vi "Control_BIn.vi"(0 "Control_1":T5={"Turbidotato 1"=1.5, "Habilitar T1"=TRUE, "Habilitar T2"=TRUE, "Habilitar T3"=TRUE, "Habilitar T4"=TRUE, "Habilitar T5"=TRUE, "Habilitar T6"=TRUE, "Habilitar T7"=TRUE, "Habilitar T8"=TRUE, "Turbidotato 2"=1.5, "Turbidotato 3"=1.5, "Turbidotato 4"=1.5, "Turbidotato 5"=1.5, "Turbidotato 6"=1.5, "Turbidotato 7"=1.5, "Turbidotato 8"=1.5, "Modo T1"=TRUE, "Modo T2"=TRUE, "Modo T3"=TRUE, "Modo T4"=TRUE, "Modo T5"=TRUE, "Modo T6"=TRUE, "Modo T7"=TRUE, "Modo T8"=TRUE} caption="Control" {"Turbidotato 8" min=0.5 max=1.5 step=0.01; "Turbidotato 7" min=0.5 max=1.5 step=0.01; "Turbidotato 6" min=0.5 max=1.5 step=0.01; "Turbidotato 5" min=0.5 max=1.5 step=0.01; "Turbidotato 4" min=0.5 max=1.5 step=0.01; "Turbidotato 3" min=0.5 max=1.5 step=0.01; "Turbidotato 2" min=0.5 max=1.5 step=0.01; "Turbidotato 1" min=0.5 max=1.5 step=0.01}, 1 "Minimos":dbl[](array[numeric]), 2 "Manual_ON":T4, 3 "Manual_Off":T3, 4 "Tiempos ON":T2={"T.M.CH1"=20, "T.M.CH2"=20, "T.M.CH3"=20, "T.M.CH4"=20, "T.M.CH5"=20, "T.M.CH6"=20, "T.M.CH7"=20, "T.M.CH8"=20} {"T.M.CH8" min=1 step=1; "T.M.CH7" min=1 step=1; "T.M.CH6" min=1 step=1; "T.M.CH5" min=1 step=1; "T.M.CH4" min=1 step=1; "T.M.CH3" min=1 step=1; "T.M.CH2" min=1 step=1; "T.M.CH1" min=1 step=1}, 5 "Tiempos OFF":T1={"T.M.CH1"=20, "T.M.CH2"=20, "T.M.CH3"=20, "T.M.CH4"=20, "T.M.CH5"=20, "T.M.CH6"=20, "T.M.CH7"=20, "T.M.CH8"=20} {"T.M.CH8" min=1 step=1; "T.M.CH7" min=1 step=1; "T.M.CH6" min=1 step=1; "T.M.CH5" min=1 step=1; "T.M.CH4" min=1 step=1; "T.M.CH3" min=1 step=1; "T.M.CH2" min=1 step=1; "T.M.CH1" min=1 step=1}, 6 "Enable Turbi?":bool, 7 "Error In":errorcluster, 8 "T-On (s)":dbl, 10 "T+ (s)":dbl=1.0 min=1.0 max=20.0) -> (20 "Estados":bool[](array[boolean]), 21 "B_OUT":bool, 27 "Error Out":errorcluster)   [LabVIEW 2013]
uses:
  Controles/Control_1_TB.ctl
  Controles/Manual_ON_TB.ctl
  Controles/Manual_OFF_TB.ctl
  Controles/Tiempos_ON_TB.ctl
  Controles/Tiempos_OFF_TB.ctl
panel:
  # "para modo Turbidostato"
  # "MODO TURBIDOSTATO"
  # "T. OFF (s)"
  # "T. ON (s)"
  # "Habilitar"
  # "Modo"
  # "CH 1"
  # "CH 2"
  # "CH 3"
  # "CH 4"
  # "CH 5"
  # "CH 6"
  # "CH 7"
  # "CH 8"
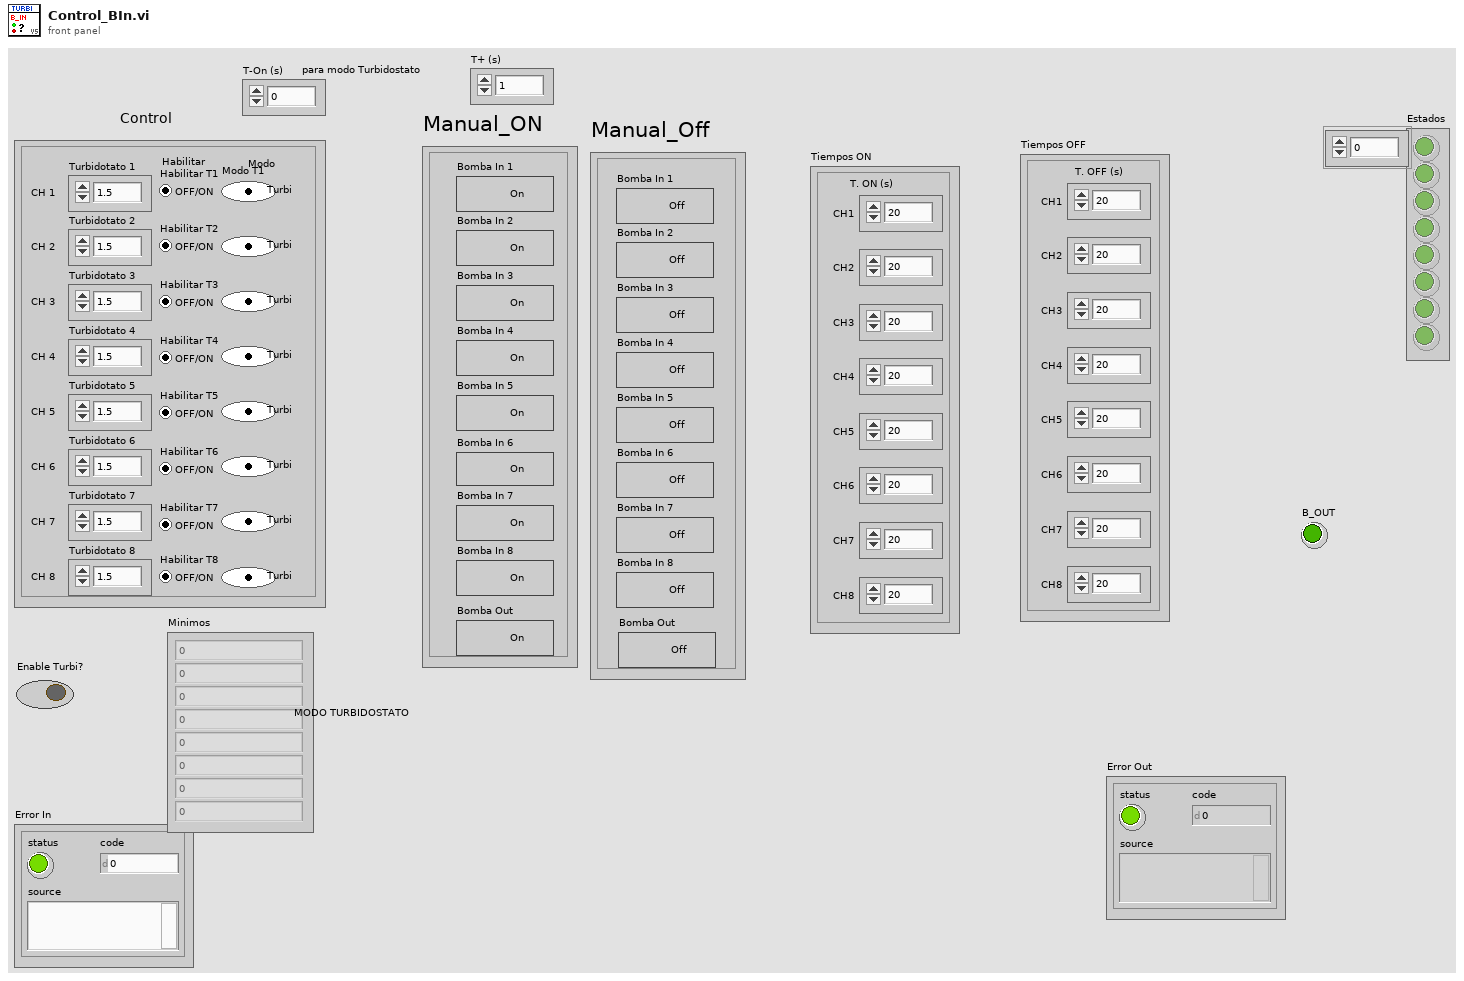
[diagram p1: front panel]
types:
  T1 = typedef "Tiempos_OFF_TB.ctl" = cluster{"T.M.CH1":u16, "T.M.CH2":u16, "T.M.CH3":u16, "T.M.CH4":u16, "T.M.CH5":u16, "T.M.CH6":u16, "T.M.CH7":u16, "T.M.CH8":u16}
  T2 = typedef "Tiempos_ON_TB.ctl" = cluster{"T.M.CH1":u16, "T.M.CH2":u16, "T.M.CH3":u16, "T.M.CH4":u16, "T.M.CH5":u16, "T.M.CH6":u16, "T.M.CH7":u16, "T.M.CH8":u16}
  T3 = typedef "Manual_OFF_TB.ctl" = cluster{"Bomba In 1-1":bool, "Bomba In 1-2":bool, "Bomba In 1-3":bool, "Bomba In 1-4":bool, "Bomba In 1-5":bool, "Bomba In 1-6":bool, "Bomba In 1-7":bool, "Bomba In 1-8":bool, "Bomba Out1":bool}
  T4 = typedef "Manual_ON_TB.ctl" = cluster{"Bomba In 1":bool, "Bomba In 2":bool, "Bomba In 3":bool, "Bomba In 4":bool, "Bomba In 5":bool, "Bomba In 6":bool, "Bomba In 7":bool, "Bomba In 8":bool, "Bomba OUT":bool}
  T5 = typedef "Control_1_TB.ctl" = cluster{"Turbidotato 1":sgl, "Habilitar T1":bool, "Habilitar T2":bool, "Habilitar T3":bool, "Habilitar T4":bool, "Habilitar T5":bool, "Habilitar T6":bool, "Habilitar T7":bool, "Habilitar T8":bool, "Turbidotato 2":sgl, "Turbidotato 3":sgl, "Turbidotato 4":sgl, "Turbidotato 5":sgl, "Turbidotato 6":sgl, "Turbidotato 7":sgl, "Turbidotato 8":sgl, "Modo T1":bool, "Modo T2":bool, "Modo T3":bool, "Modo T4":bool, "Modo T5":bool, "Modo T6":bool, "Modo T7":bool, "Modo T8":bool}
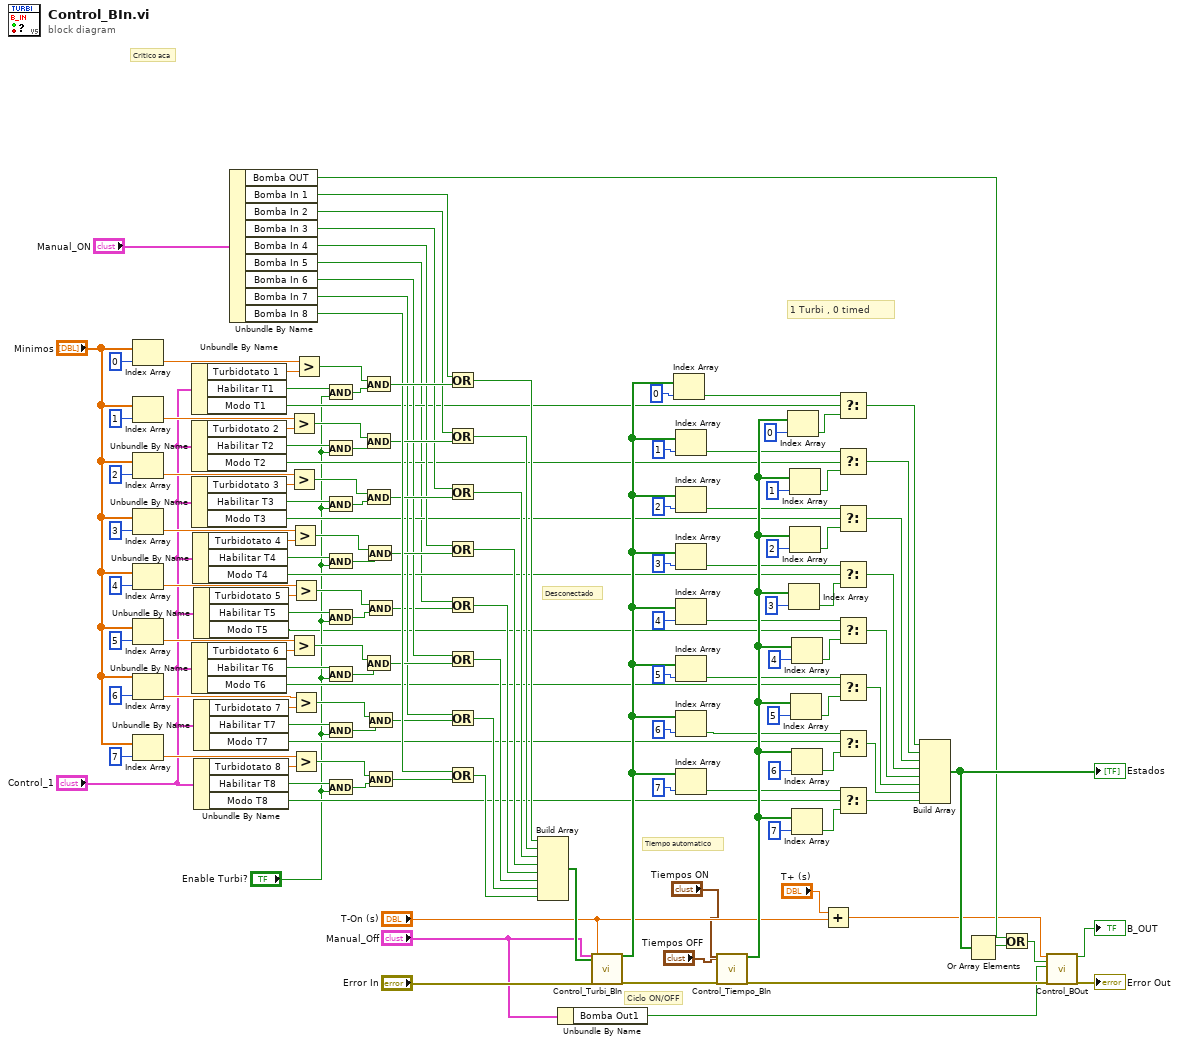
[diagram p0: block diagram]
diagram:
  # "Desconectado"
  # "1 Turbi , 0 timed"
  # "Critico aca"
  # "Ciclo ON/OFF"
  # "Tiempo automatico"
  n1 = Index Array(array="Minimos", index=0) -> (element=w134:dbl)
  n2 = Index Array(array="Minimos", index=1) -> (element=w117:dbl)
  n3 = Index Array(array="Minimos", index=2) -> (element=w116:dbl)
  n4 = Index Array(array="Minimos", index=3) -> (element=w115:dbl)
  n5 = Index Array(array="Minimos", index=4) -> (element=w114:dbl)
  n6 = Index Array(array="Minimos", index=5) -> (element=w113:dbl)
  n7 = Index Array(array="Minimos", index=6) -> (element=w112:dbl)
  n8 = Index Array(array="Minimos", index=7) -> (element=w111:dbl)
  n9 = Unbundle By Name("Control_1") -> ("Turbidotato 1"=w133:sgl, "Habilitar T1"=w21:bool, "Modo T1"=w63:bool)
  n10 = Unbundle By Name("Control_1") -> ("Turbidotato 2"=w130:sgl, "Habilitar T2"=w12:bool, "Modo T2"=w60:bool)
  n11 = Unbundle By Name("Control_1") -> ("Turbidotato 3"=w129:sgl, "Habilitar T3"=w11:bool, "Modo T3"=w59:bool)
  n12 = Unbundle By Name("Control_1") -> ("Turbidotato 6"=w122:sgl, "Habilitar T6"=w8:bool, "Modo T6"=w52:bool)
  n13 = Unbundle By Name("Control_1") -> ("Turbidotato 4"=w126:sgl, "Habilitar T4"=w10:bool, "Modo T4"=w56:bool)
  n14 = Unbundle By Name("Control_1") -> ("Turbidotato 5"=w125:sgl, "Habilitar T5"=w9:bool, "Modo T5"=w1:bool)
  n15 = Unbundle By Name("Control_1") -> ("Turbidotato 7"=w121:sgl, "Habilitar T7"=w7:bool, "Modo T7"=w51:bool)
  n16 = Unbundle By Name("Control_1") -> ("Turbidotato 8"=w118:sgl, "Habilitar T8"=w14:bool, "Modo T8"=w61:bool)
  n17 = Unbundle By Name("Manual_ON") -> ("Bomba OUT"=w29:bool, "Bomba In 1"=w85:bool, "Bomba In 2"=w77:bool, "Bomba In 3"=w76:bool, "Bomba In 4"=w75:bool, "Bomba In 5"=w3:bool, "Bomba In 6"=w74:bool, "Bomba In 7"=w73:bool, "Bomba In 8"=w83:bool)
  n18 = Greater?(x=w117, y=w130) -> (0:w131:bool)
  n19 = Greater?(x=w116, y=w129) -> (0:w128:bool)
  n20 = Greater?(x=w113, y=w122) -> (0:w123:bool)
  n21 = Greater?(x=w115, y=w126) -> (0:w127:bool)
  n22 = Greater?(x=w114, y=w125) -> (0:w124:bool)
  n23 = Greater?(x=w112, y=w121) -> (0:w120:bool)
  n24 = Greater?(x=w111, y=w118) -> (0:w119:bool)
  n25 = Greater?(x=w134, y=w133) -> (0:w132:bool)
  n26 = And(x=w21, y="Enable Turbi?") -> (x .and. y?=w22:bool)
  n27 = And(x=w12, y="Enable Turbi?") -> (x .and. y?=w20:bool)
  n28 = And(x=w11, y="Enable Turbi?") -> (x .and. y?=w19:bool)
  n29 = And(x=w10, y="Enable Turbi?") -> (x .and. y?=w18:bool)
  n30 = And(x=w9, y="Enable Turbi?") -> (x .and. y?=w17:bool)
  n31 = And(x=w8, y="Enable Turbi?") -> (x .and. y?=w16:bool)
  n32 = And(x=w7, y="Enable Turbi?") -> (x .and. y?=w15:bool)
  n33 = And(x=w14, y="Enable Turbi?") -> (x .and. y?=w13:bool)
  n34 = And(x=w132, y=w22) -> (x .and. y?=w86:bool)
  n35 = And(x=w131, y=w20) -> (x .and. y?=w82:bool)
  n36 = And(x=w128, y=w19) -> (x .and. y?=w81:bool)
  n37 = And(x=w123, y=w16) -> (x .and. y?=w79:bool)
  n38 = And(x=w127, y=w18) -> (x .and. y?=w80:bool)
  n39 = And(x=w124, y=w17) -> (x .and. y?=w2:bool)
  n40 = And(x=w120, y=w15) -> (x .and. y?=w78:bool)
  n41 = And(x=w119, y=w13) -> (x .and. y?=w84:bool)
  n42 = Or(x=w85, y=w86) -> (x .or. y?=w70:bool)
  n43 = Or(x=w77, y=w82) -> (x .or. y?=w69:bool)
  n44 = Or(x=w76, y=w81) -> (x .or. y?=w68:bool)
  n45 = Or(x=w75, y=w80) -> (x .or. y?=w67:bool)
  n46 = Or(x=w3, y=w2) -> (x .or. y?=w66:bool)
  n47 = Or(x=w74, y=w79) -> (x .or. y?=w65:bool)
  n48 = Or(x=w73, y=w78) -> (x .or. y?=w64:bool)
  n49 = Or(x=w83, y=w84) -> (x .or. y?=w71:bool)
  n50 = Build Array(w70, w69, w68, w67, w66, w65, w64, w71) -> (w72:bool[])
  n51 = Unbundle By Name("Manual_Off") -> ("Bomba Out1"=w25:bool)
  n52 = call "Control_Turbi_BIn.vi"("Manual_Off"="Manual_Off", "Estados_IN"=w72, "Error In"="Error In", "T-On (s)"="T-On (s)") -> ("Estados_OUT"=w89:bool[], "Error Out"=w99:errorcluster)  [unwired: 22 in]
  n53 = Index Array(array=w89, index=0) -> (element=w88:bool)
  n54 = Index Array(array=w89, index=1) -> (element=w58:bool)
  n55 = Index Array(array=w89, index=2) -> (element=w57:bool)
  n56 = Index Array(array=w89, index=3) -> (element=w55:bool)
  n57 = Index Array(array=w89, index=4) -> (element=w54:bool)
  n58 = Index Array(array=w89, index=5) -> (element=w49:bool)
  n59 = Index Array(array=w89, index=6) -> (element=w50:bool)
  n60 = Index Array(array=w89, index=7) -> (element=w53:bool)
  n61 = call "Control_Tiempo_BIn.vi"("Tiempos ON"="Tiempos ON", "Tiempos OFF"="Tiempos OFF", "error in"=w99) -> ("Estados_Salidas"=w100:bool[], "Error Out"=w28:errorcluster)  [unwired: 15 in]
  n62 = Index Array(array=w100, index=0) -> (element=w62:bool)
  n63 = Index Array(array=w100, index=3) -> (element=w46:bool)
  n64 = Index Array(array=w100, index=1) -> (element=w48:bool)
  n65 = Index Array(array=w100, index=2) -> (element=w47:bool)
  n66 = Index Array(array=w100, index=5) -> (element=w44:bool)
  n67 = Index Array(array=w100, index=4) -> (element=w45:bool)
  n68 = Index Array(array=w100, index=6) -> (element=w43:bool)
  n69 = Index Array(array=w100, index=7) -> (element=w42:bool)
  n70 = Add(x="T+ (s)", y="T-On (s)") -> (x+y=w26:dbl)
  n71 = Select(t=w88, s=w63, f=w62) -> (s? t:f=w87:bool)
  n72 = Select(t=w58, s=w60, f=w48) -> (s? t:f=w40:bool)
  n73 = Select(t=w57, s=w59, f=w47) -> (s? t:f=w39:bool)
  n74 = Select(t=w55, s=w56, f=w46) -> (s? t:f=w38:bool)
  n75 = Select(t=w54, s=w1, f=w45) -> (s? t:f=w37:bool)
  n76 = Select(t=w49, s=w52, f=w44) -> (s? t:f=w36:bool)
  n77 = Select(t=w50, s=w51, f=w43) -> (s? t:f=w35:bool)
  n78 = Select(t=w53, s=w61, f=w42) -> (s? t:f=w41:bool)
  n79 = Build Array(w87, w40, w39, w38, w37, w36, w35, w41) -> (w34:bool[])
  "Estados" <- w34
  n80 = Or Array Elements(Boolean array=w34) -> (logical OR=w30:bool)
  n81 = Or(x=w29, y=w30) -> (x .or. y?=w27:bool)
  n82 = call "Control_BOut.vi"("T-On (s)"=w26, "Estado"=w27, "Off Manual"=w25, "Error In"=w28) -> ("Estado_OUT"=→"B_OUT":bool, "Error Out"=→"Error Out":errorcluster)  [unwired: 14 in]
